vi "Setup.vi"(11 "TEMPLATE Actor in":refnum<class "{{Name}}Actor.lvclass">) -> (0 "Error out":errorcluster, 3 "TEMPLATE Actor out":refnum<class "{{Name}}Actor.lvclass">)   [LabVIEW 2020, in "_Template.lvlib" / "Templates.lvlib" / "{{Name}}Actor.lvlib" / "{{Name}}Actor.lvclass"]
uses:
  {{Name}}Actor.lvclass
  {{Name}}Actor.lvclass/{{Name}}Actor.ctl
  jettl/jettl/Actor/Actor.lvclass
panel:
  # "This front panel should not be manipulated."
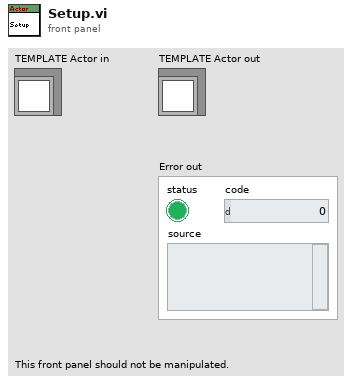
[diagram p1: front panel]
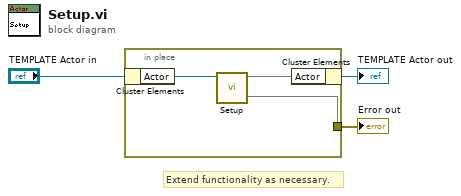
[diagram p0: block diagram]
diagram:
  # "Extend functionality as necessary."
  n1 = in-place {
    in-place-border: [w6] -> w1
    n2 = in-place-cluster #1("TEMPLATE Actor in") -> ("Actor"=w5:refnum<class "Actor.lvclass">)
    n3 = call-dynamic "Setup.vi"(11:w5) -> (0:w6, 3:w4)  [unwired: 7 in, 2 out]
    n4 = in-place-cluster #1("Actor"=w4) -> (→"TEMPLATE Actor out":refnum<class "{{Name}}Actor.lvclass">)
  }
  "Error out" <- w1
